vi "Übertragung.vi"() -> ()   [LabVIEW 2017]
uses:
  <vilib>/Instr/_visa.llb/VISA Configure Serial Port (Instr).vi
panel:
  in  "Anzahl Ventilplatine":i32
  out "startbereit ?":bool
  in  "manuell Starten":bool
  in  "starten":bool
  in  "Messtabelle":dbl[][](array[numeric])
  in  "Messaufloesung":i32
  in  "Baudrate":dbl
  in  "Com":refnum<visa-resource-name> caption="VISA-Ressourcenname"
  in  "Header":string[][](array[string])
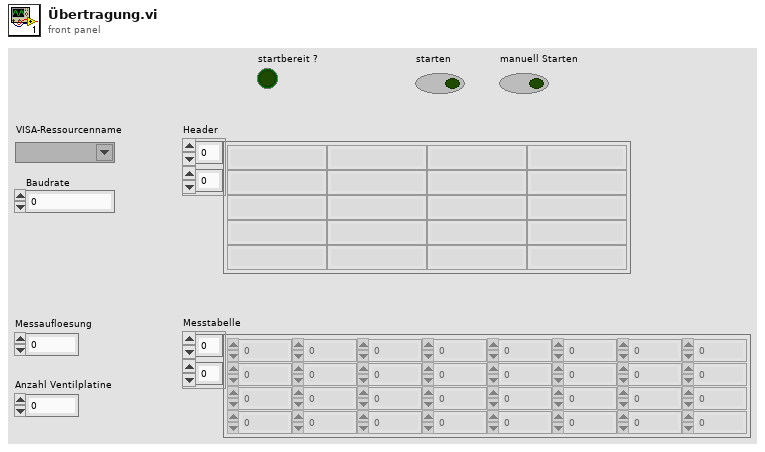
[diagram p1: front panel]
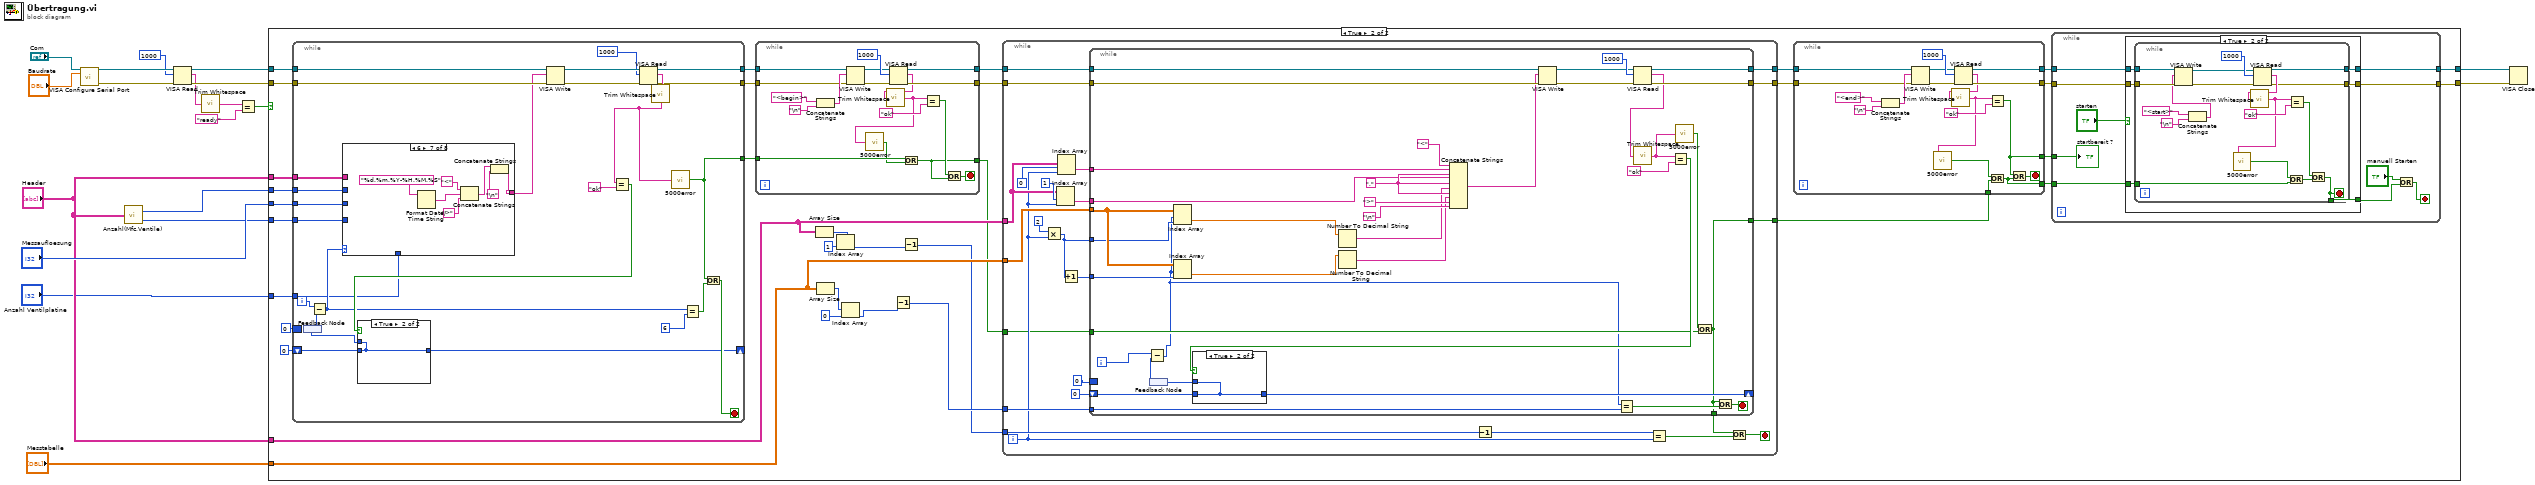
[diagram p0: block diagram]
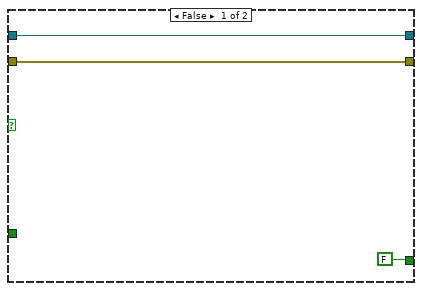
[diagram p3: hidden frame]
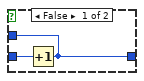
[diagram p4: hidden frame]
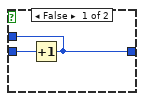
[diagram p5: hidden frame]
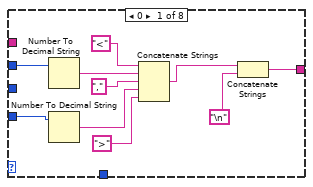
[diagram p6: hidden frame]
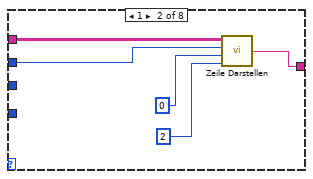
[diagram p7: hidden frame]
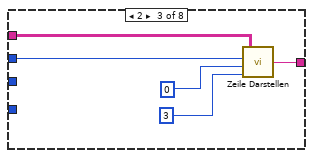
[diagram p8: hidden frame]
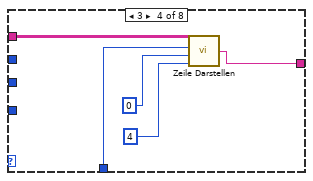
[diagram p9: hidden frame]
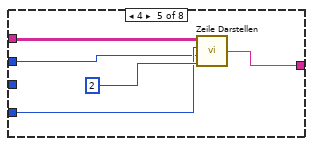
[diagram p10: hidden frame]
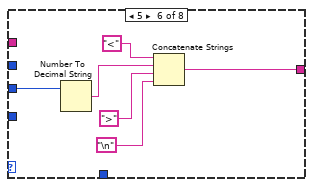
[diagram p11: hidden frame]
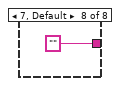
[diagram p12: hidden frame]
diagram:
  n1 = call-poly "VISA Configure Serial Port"("VISA resource name"="Com", "baud rate (9600)"="Baudrate") -> ("VISA resource name out"=w18:refnum<visa-resource-name>, "error out"=w17:errorcluster)  [unwired: 12 in]
  n2 = call "Anzahl(Mfc,Ventile).vi"("Array"="Header") -> ("Anzahal Mfc's"=w19:i32, "Anzahl Ventile"=w1:i32)
  n3 = VISA Read(VISA resource name=w18, byte count=1000, error in (no error)=w17) -> (VISA resource name out=w12:refnum<visa-resource-name>, read buffer=w10:string, error out=w11:errorcluster)  [unwired: 1 out]
  n4 = call <vilib>:"Trim Whitespace.vi"("string"=w10) -> ("trimmed string"=w9:string)  [unwired: 1 in]
  n5 = Equal?(x=w9, y="ready") -> (x = y?=w6:bool)
  n6 = case shown="True" w6 {
    tunnel: w19 -> [_ w55]
    tunnel: "Header" -> [_ w54]
    tunnel: w12 -> [w20 w53]
    tunnel: w11 -> [w21 w52]
    tunnel: [w20 w33] -> w16
    tunnel: [w21 w32] -> w15
    tunnel: "Messaufloesung" -> [_ w49]
    tunnel: "Messtabelle" -> [_ w44]
    tunnel: "Header" -> [_ w39]
    tunnel: "Anzahl Ventilplatine" -> [_ w27]
    tunnel: w1 -> [_ w26]
    frame False {
    }
    frame True {
      n7 = while {
        tunnel: w55 -> [w219]
        tunnel: w54 -> [w218]
        tunnel: w53 -> [w217]
        tunnel: w52 -> [w216]
        shift-right: [w202] -> _
        shift-left: 0 -> [w209]
        tunnel: [w207] -> w51
        tunnel: [w206] -> w50
        tunnel: w49 -> [w200]
        tunnel: [w196] -> w38
        border: 0 -> [_]
        tunnel: w27 -> [w195]
        tunnel: w26 -> [w194]
        i -> [w208]
        stop <- w211 stop-if-true
        n8 = feedback #1() -> (w197:i32)
        n9 = Subtract(x=w208, y=w197) -> (x-y=w199:i32)
        n10 = case shown="6" w199 {
          tunnel: [w224 w237 w239 w245 w250 w256 w260 ""] -> w193
          tunnel: w219 -> [w231 w233 w238 _ w248 _ _ _]
          tunnel: w218 -> [_ w236 w242 w243 w252 _ _ _]
          tunnel: w200 -> [_ _ _ _ _ w258 _ _]
          tunnel: w195 -> [_ _ _ w244 _ _ _ _]
          tunnel: w194 -> [w223 _ _ _ w249 _ _ _]
          frame 0 {
            n11 = Number To Decimal String(number=w231) -> (decimal integer string=w230:string)  [unwired: 1 in]
            n12 = Number To Decimal String(number=w223) -> (decimal integer string=w229:string)  [unwired: 1 in]
            n13 = Concatenate Strings("<", w230, ",", w229, ">") -> (w225:string)
            n14 = Concatenate Strings(w225, "\n") -> (w224:string)
          }
          frame 1 {
            n15 = call "Zeile Darstellen.vi"("Zeile"=2, "Anfangsspalte"=0, "Anzahl der Elemnte"=w233, "Array"=w236) -> ("String"=w237:string)
          }
          frame 2 {
            n16 = call "Zeile Darstellen.vi"("Zeile"=3, "Anfangsspalte"=0, "Anzahl der Elemnte"=w238, "Array"=w242) -> ("String"=w239:string)
          }
          frame 3 {
            n17 = call "Zeile Darstellen.vi"("Zeile"=4, "Anfangsspalte"=0, "Anzahl der Elemnte"=w244, "Array"=w243) -> ("String"=w245:string)
          }
          frame 4 {
            n18 = call "Zeile Darstellen.vi"("Zeile"=2, "Anfangsspalte"=w248, "Anzahl der Elemnte"=w249, "Array"=w252) -> ("String"=w250:string)
          }
          frame 5 {
            n19 = Number To Decimal String(number=w258) -> (decimal integer string=w255:string)  [unwired: 1 in]
            n20 = Concatenate Strings("<", w255, ">", "\n") -> (w256:string)
          }
          frame 6 {
            n21 = Format Date/Time String(time format string (%c)="%d.%m.%Y-%H.%M.%S") -> (date/time string=w265:string)  [unwired: 2 in]
            n22 = Concatenate Strings("<", w265, ">") -> (w259:string)
            n23 = Concatenate Strings(w259, "\n") -> (w260:string)
          }
          frame 7, Default {
          }
        }
        n24 = VISA Write(VISA resource name=w217, write buffer=w193, error in (no error)=w216) -> (VISA resource name out=w215:refnum<visa-resource-name>, error out=w214:errorcluster)  [unwired: 1 out]
        n25 = VISA Read(VISA resource name=w215, byte count=1000, error in (no error)=w214) -> (VISA resource name out=w207:refnum<visa-resource-name>, read buffer=w212:string, error out=w206:errorcluster)  [unwired: 1 out]
        n26 = call <vilib>:"Trim Whitespace.vi"("string"=w212) -> ("trimmed string"=w201:string)  [unwired: 1 in]
        n27 = Equal?(x=w201, y="ok") -> (x = y?=w210:bool)
        n28 = case shown="True" w210 {
          tunnel: w209 -> [w221 w222]
          tunnel: [w220 w222] -> w198
          tunnel: [w220 w222] -> w202
          frame False {
            n29 = Increment(x=w221) -> (x+1=w220:i32)
          }
          frame True {
          }
        }
        n30 = feedback-in #1(w198) -> ()
        n31 = call "5000error.vi"("String"=w201) -> ("x UND y?"=w196:bool)
        n32 = Equal?(x=w199, y=6) -> (x = y?=w204:bool)
        n33 = Or(x=w196, y=w204) -> (x .or. y?=w211:bool)
      }
      n34 = while {
        tunnel: w51 -> [w188]
        tunnel: [w186] -> w43
        tunnel: w50 -> [w185]
        tunnel: [w183] -> w42
        tunnel: w38 -> [w177]
        tunnel: [w175] -> w37
        stop <- w178 stop-if-true
        n35 = Concatenate Strings("<begin>", "\n") -> (w190:string)
        n36 = VISA Write(VISA resource name=w188, write buffer=w190, error in (no error)=w185) -> (VISA resource name out=w187:refnum<visa-resource-name>, error out=w184:errorcluster)  [unwired: 1 out]
        n37 = VISA Read(VISA resource name=w187, byte count=1000, error in (no error)=w184) -> (VISA resource name out=w186:refnum<visa-resource-name>, read buffer=w181:string, error out=w183:errorcluster)  [unwired: 1 out]
        n38 = call <vilib>:"Trim Whitespace.vi"("string"=w181) -> ("trimmed string"=w180:string)  [unwired: 1 in]
        n39 = call "5000error.vi"("String"=w180) -> ("x UND y?"=w176:bool)
        n40 = Or(x=w177, y=w176) -> (x .or. y?=w175:bool)
        n41 = Equal?(x=w180, y="ok") -> (x = y?=w179:bool)
        n42 = Or(x=w179, y=w175) -> (x .or. y?=w178:bool)
      }
      n43 = Array Size(array=w39) -> (size(s)=w46:i32[])
      n44 = Array Size(array=w44) -> (size(s)=w48:i32[])
      n45 = Index Array(array=w46, index=1) -> (element=w23:i32)
      n46 = Index Array(array=w48, index=0) -> (element=w25:i32)
      n47 = Decrement(x=w25) -> (x-1=w24:i32)
      n48 = Decrement(x=w23) -> (x-1=w22:i32)
      n49 = while {
        tunnel: w24 -> [w103]
        tunnel: w44 -> [w112]
        tunnel: w22 -> [w109]
        tunnel: w43 -> [w108]
        tunnel: w42 -> [w107]
        tunnel: [w106] -> w41
        tunnel: [w105] -> w40
        tunnel: w39 -> [w102]
        tunnel: w37 -> [w95]
        tunnel: [w94] -> w36
        i -> [w100]
        stop <- w96 stop-if-true
        n50 = Multiply(x=2, y=w100) -> (x*y=w111:i32)
        n51 = Index Array(array=w102, index (row)=1, index (col)=w100) -> (element=w113:string)
        n52 = Index Array(array=w102, index (row)=0, index (col)=w100) -> (element=w114:string)
        n53 = Increment(x=w111) -> (x+1=w110:i32)
        n54 = while {
          tunnel: w114 -> [w147]
          tunnel: w113 -> [w146]
          tunnel: w112 -> [w145]
          tunnel: w111 -> [w144]
          tunnel: w110 -> [w143]
          tunnel: w108 -> [w140]
          tunnel: w107 -> [w139]
          tunnel: [w138] -> w106
          tunnel: [w137] -> w105
          shift-right: [w133] -> _
          shift-left: 0 -> [w134]
          tunnel: w103 -> [w132]
          tunnel: [w121] -> w98
          tunnel: w95 -> [w122]
          tunnel: [w121] -> w94
          border: 0 -> [_]
          i -> [w119]
          stop <- w130 stop-if-true
          w152 = ","
          n55 = feedback #2() -> (w117:i32)
          n56 = Subtract(x=w119, y=w117) -> (x-y=w120:i32)
          n57 = Index Array(array=w145, index (row)=w120, index (col)=w144) -> (element=w142:dbl)
          n58 = Index Array(array=w145, index (row)=w120, index (col)=w143) -> (element=w141:dbl)
          n59 = Number To Decimal String(number=w142) -> (decimal integer string=w149:string)  [unwired: 1 in]
          n60 = Number To Decimal String(number=w141) -> (decimal integer string=w148:string)  [unwired: 1 in]
          n61 = Concatenate Strings("<", w147, w152, w146, w152, w149, w152, w148, ">", "\n") -> (w129:string)
          n62 = VISA Write(VISA resource name=w140, write buffer=w129, error in (no error)=w139) -> (VISA resource name out=w128:refnum<visa-resource-name>, error out=w127:errorcluster)  [unwired: 1 out]
          n63 = Equal?(x=w120, y=w132) -> (x = y?=w131:bool)
          n64 = VISA Read(VISA resource name=w128, byte count=1000, error in (no error)=w127) -> (VISA resource name out=w138:refnum<visa-resource-name>, read buffer=w125:string, error out=w137:errorcluster)  [unwired: 1 out]
          n65 = call <vilib>:"Trim Whitespace.vi"("string"=w125) -> ("trimmed string"=w126:string)  [unwired: 1 in]
          n66 = Equal?(x=w126, y="ok") -> (x = y?=w124:bool)
          n67 = case shown="True" w124 {
            tunnel: [w154 w156] -> w118
            tunnel: [w154 w156] -> w133
            tunnel: w134 -> [w155 w156]
            frame False {
              n68 = Increment(x=w155) -> (x+1=w154:i32)
            }
            frame True {
            }
          }
          n69 = feedback-in #2(w118) -> ()
          n70 = call "5000error.vi"("String"=w126) -> ("x UND y?"=w123:bool)
          n71 = Or(x=w123, y=w122) -> (x .or. y?=w121:bool)
          n72 = Or(x=w121, y=w131) -> (x .or. y?=w130:bool)
        }
        n73 = Decrement(x=w109) -> (x-1=w99:i32)
        n74 = Equal?(x=w99, y=w100) -> (x = y?=w97:bool)
        n75 = Or(x=w98, y=w97) -> (x .or. y?=w96:bool)
      }
      n76 = while {
        tunnel: w41 -> [w170]
        tunnel: [w168] -> w30
        tunnel: w40 -> [w167]
        tunnel: [w165] -> w31
        tunnel: w36 -> [w159]
        tunnel: [w158] -> w29
        tunnel: [w157] -> w28
        stop <- w161 stop-if-true
        n77 = Concatenate Strings("<end>", "\n") -> (w172:string)
        n78 = VISA Write(VISA resource name=w170, write buffer=w172, error in (no error)=w167) -> (VISA resource name out=w169:refnum<visa-resource-name>, error out=w166:errorcluster)  [unwired: 1 out]
        n79 = VISA Read(VISA resource name=w169, byte count=1000, error in (no error)=w166) -> (VISA resource name out=w168:refnum<visa-resource-name>, read buffer=w163:string, error out=w165:errorcluster)  [unwired: 1 out]
        n80 = call <vilib>:"Trim Whitespace.vi"("string"=w163) -> ("trimmed string"=w162:string)  [unwired: 1 in]
        n81 = call "5000error.vi"("String"=w162) -> ("x UND y?"=w160:bool)
        n82 = Or(x=w160, y=w159) -> (x .or. y?=w158:bool)
        n83 = Equal?(x=w162, y="ok") -> (x = y?=w157:bool)
        n84 = Or(x=w157, y=w158) -> (x .or. y?=w161:bool)
      }
      n85 = while {
        tunnel: w29 -> [w61]
        tunnel: w31 -> [w63]
        tunnel: [w64] -> w32
        tunnel: w30 -> [w62]
        tunnel: [w65] -> w33
        tunnel: w28 -> [w56]
        stop <- w57 stop-if-true
        n86 = case shown="True" "starten" {
          tunnel: [w68 w74] -> w65
          tunnel: [w67 w73] -> w64
          tunnel: w63 -> [w67 w72]
          tunnel: w62 -> [w68 w71]
          tunnel: w61 -> [_ w70]
          tunnel: [FALSE w69] -> w58
          frame False {
          }
          frame True {
            n87 = while {
              tunnel: [w78] -> w74
              tunnel: [w77] -> w73
              tunnel: w72 -> [w92]
              tunnel: w71 -> [w91]
              tunnel: w70 -> [w76]
              tunnel: [w75] -> w69
              stop <- w75 stop-if-true
              n88 = Concatenate Strings("<start>", "\n") -> (w88:string)
              n89 = VISA Write(VISA resource name=w91, write buffer=w88, error in (no error)=w92) -> (VISA resource name out=w80:refnum<visa-resource-name>, error out=w79:errorcluster)  [unwired: 1 out]
              n90 = VISA Read(VISA resource name=w80, byte count=1000, error in (no error)=w79) -> (VISA resource name out=w78:refnum<visa-resource-name>, read buffer=w85:string, error out=w77:errorcluster)  [unwired: 1 out]
              n91 = call <vilib>:"Trim Whitespace.vi"("string"=w85) -> ("trimmed string"=w84:string)  [unwired: 1 in]
              n92 = call "5000error.vi"("String"=w84) -> ("x UND y?"=w82:bool)
              n93 = Or(x=w82, y=w76) -> (x .or. y?=w81:bool)
              n94 = Equal?(x=w84, y="ok") -> (x = y?=w83:bool)
              n95 = Or(x=w83, y=w81) -> (x .or. y?=w75:bool)
            }
          }
        }
        n96 = Or(x="manuell Starten", y=w58) -> (x .or. y?=w57:bool)
        "startbereit ?" <- w56
      }
    }
  }
  n97 = VISA Close(VISA resource name=w16, error in (no error)=w15) -> ()  [unwired: 1 out]
